vi "Perform Action.vi"(8 "error in (no error)":errorcluster, 10 "Input":variant, 11 "Virtual Voltage Reader in":refnum<class "Virtual Voltage Reader.lvclass">) -> (0 "error out":errorcluster, 2 "Output":variant, 3 "Virtual Voltage Reader out":refnum<class "Virtual Voltage Reader.lvclass">)   [LabVIEW 2023, in "Scope Base.lvlib" / "Virtual Voltage Reader.lvclass"]
uses:
  Virtual Voltage Reader.lvclass
  Interfaces/IInstrument/IInstrument.lvclass
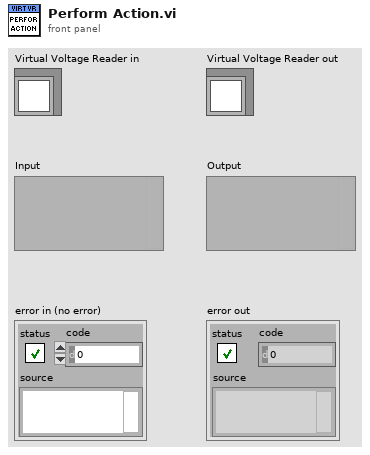
[diagram p1: front panel]
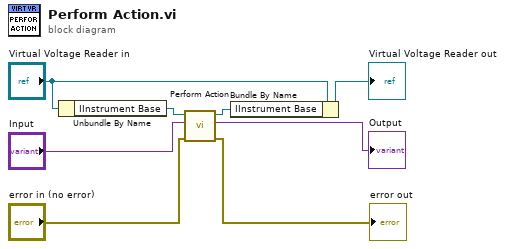
[diagram p0: block diagram]
diagram:
  n1 = Unbundle By Name("Virtual Voltage Reader in") -> ("IInstrument Base"=w8:refnum<class "IInstrument.lvclass">)
  n2 = call-dynamic "Perform Action.vi"("Error In"="error in (no error)", "Input"="Input", "object in"=w8) -> ("Error Out"=→"error out":errorcluster, "Output"=→"Output":variant, "object out"=w3:refnum<class "IInstrument.lvclass">)  [unwired: 6 in]
  n3 = Bundle By Name(cluster="Virtual Voltage Reader in", "IInstrument Base"=w3) -> (→"Virtual Voltage Reader out":refnum<class "Virtual Voltage Reader.lvclass">)
